vi "剖面数据拆分切割.vi"(11 "剖面多参数输入":string[][](array[string])) -> (3 "剖面多参数输出":string[][][](array[string]))   [LabVIEW 2016, in "数据传输系统-02.lvlib"]
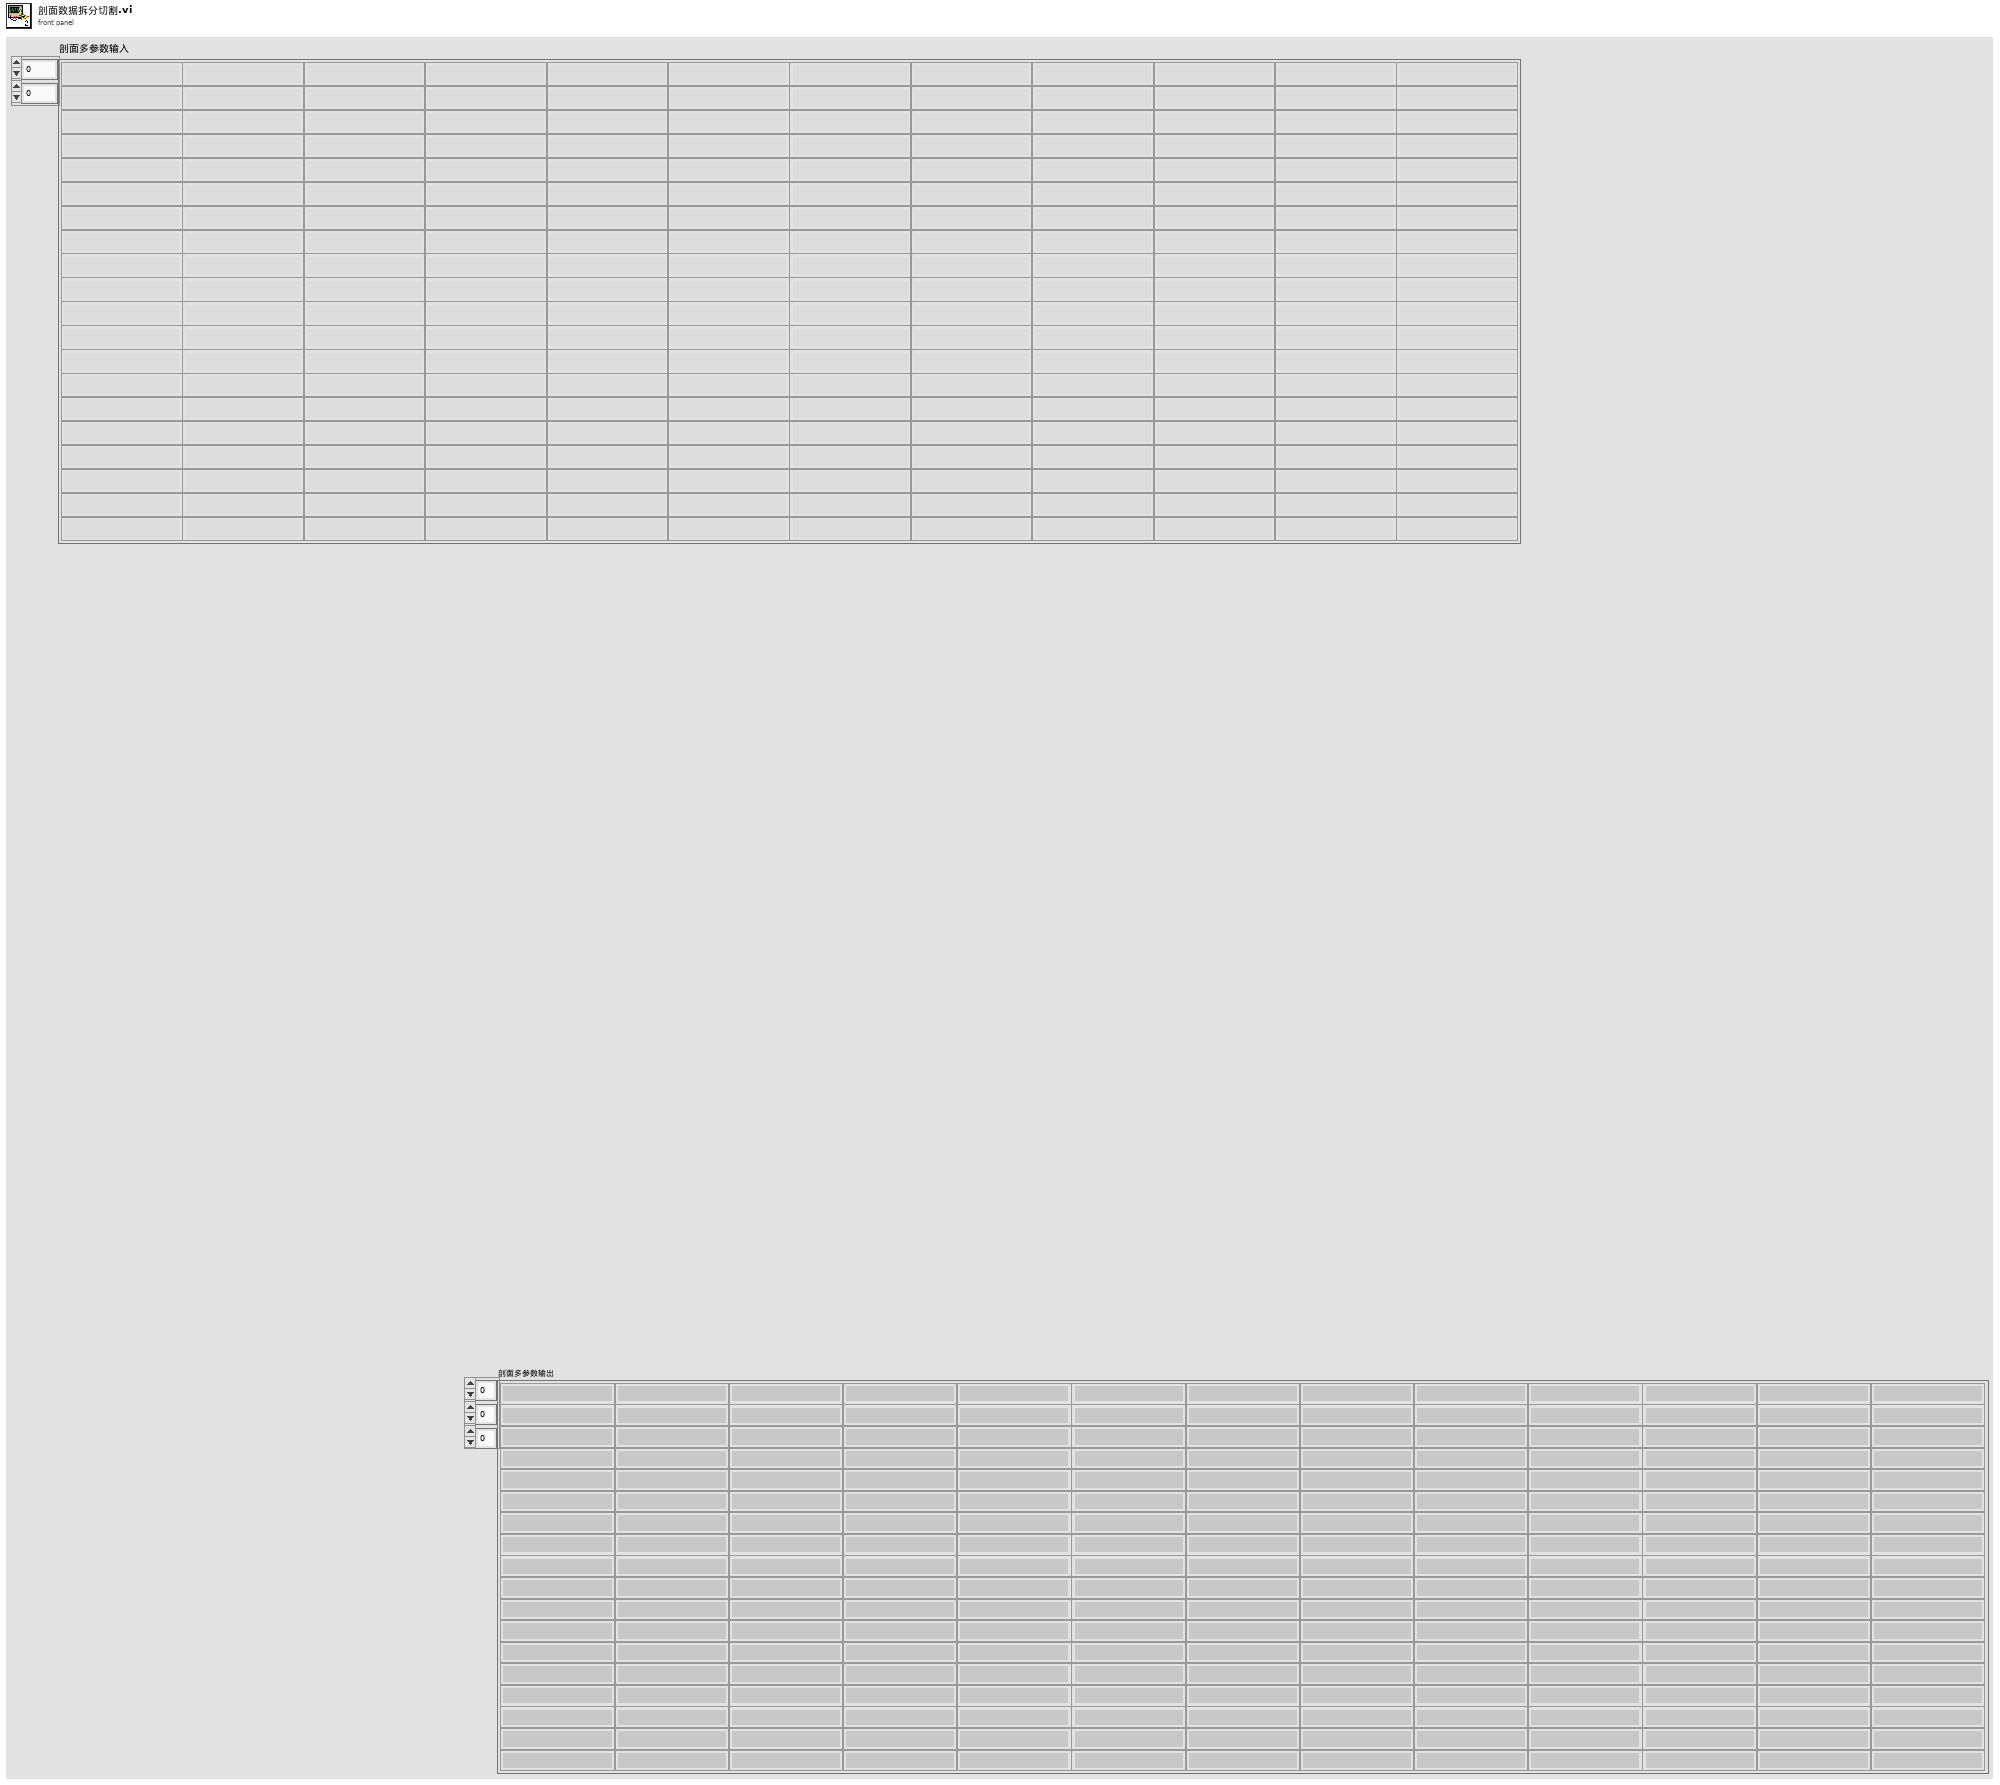
[diagram p1: front panel]
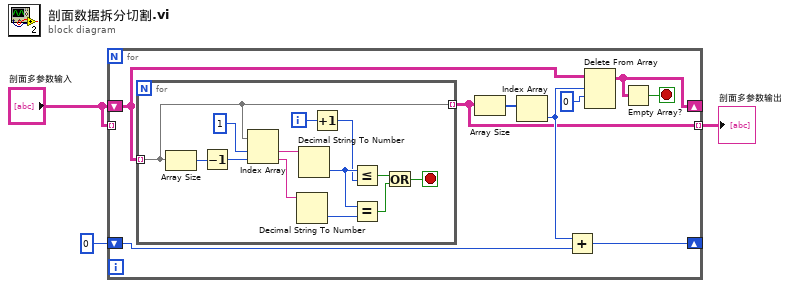
[diagram p0: block diagram]
diagram:
  n1 = for {
    shift-right: [w4] -> _
    shift-left: "剖面多参数输入" -> [w5]
    shift-right: [w9] -> _
    shift-left: 0 ("索引 (行)") -> [w10]
    tunnel: "剖面多参数输入" -> [_] mode=indexing
    tunnel: [w7] -> w2 mode=indexing
    stop <- w8 stop-if-true
    n2 = for {
      tunnel: w5 -> [w18] mode=indexing
      tunnel: [w18] -> w7 mode=indexing
      i -> [w16]
      stop <- w17 stop-if-true
      n3 = Array Size(array=w18) -> (size(s)=w24:i32)
      n4 = Decrement(x=w24) -> (x-1=w23:i32)
      n5 = Index Array(array=w18, index #1=1 ("索引"), index #2=w23) -> (element #1=w22:string, element #2=w21:string)
      n6 = Decimal String To Number(string=w21) -> (number=w20:i32)  [unwired: 2 in, 1 out]
      n7 = Decimal String To Number(string=w22) -> (number=w15:i32)  [unwired: 2 in, 1 out]
      n8 = Increment(x=w16) -> (x+1=w14:i32)
      n9 = Less Or Equal?(x=w15, y=w14) -> (x <= y?=w13:bool)
      n10 = Equal?(x=w15, y=w20) -> (x = y?=w19:bool)
      n11 = Or(x=w13, y=w19) -> (x .or. y?=w17:bool)
    }
    n12 = Array Size(array=w7) -> (size(s)=w12:i32[])
    n13 = Index Array(array=w12) -> (element=w11:i32)  [unwired: 1 in]
    n14 = Add(x=w11, y=w10) -> (x+y=w9:i32)
    n15 = Delete From Array(array=w5, length=w11, index (row)=0 ("索引 (行)")) -> (array with subset deleted=w4:string[][])  [unwired: 1 in, 1 out]
    n16 = Empty Array?(array=w4) -> (empty?=w8:bool)
  }
  "剖面多参数输出" <- w2
